vi "Help.About.vi"(11 "SW Version":T1={"AppName"="Automated Test Station", "Company"="Kwest Engineering", "Version"="v1.0.1", "Description"="1/25/2016"}) -> ()   [LabVIEW 2017]
uses:
  <vilib>/KATE/Module/Module.SW Version Info.ctl
  <vilib>/KATE/Module/Module Utils.lvlib
panel:
  in  "Close":bool
  out "About this Application:":string
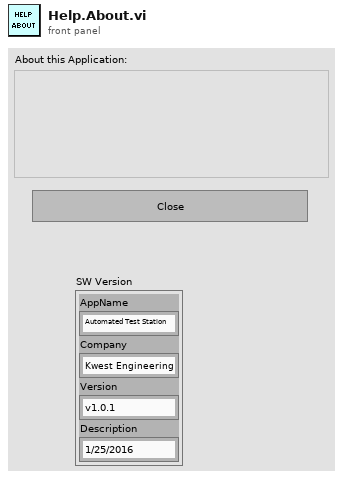
[diagram p1: front panel]
types:
  T1 = typedef "KATE_Lib.lvlib/Module Utils.lvlib/Module.SW Version Info.ctl" = cluster{"AppName":string, "Company":string, "Version":string, "Description":string}
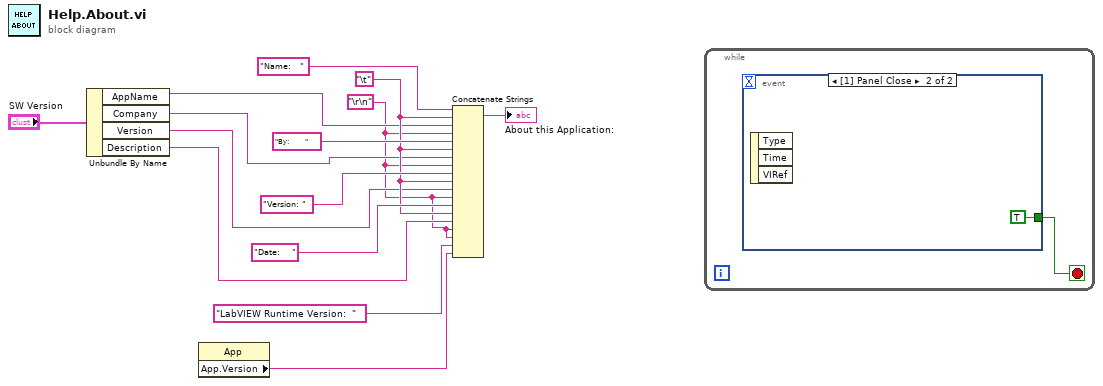
[diagram p0: block diagram]
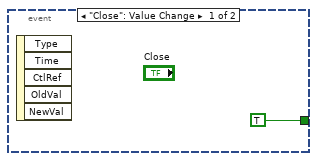
[diagram p2: hidden frame]
diagram:
  w3 = "\r\n"
  w9 = "\t"
  n1 = Unbundle By Name("SW Version") -> ("AppName"=w7:string, "Company"=w6:string, "Version"=w5:string, "Description"=w4:string)
  n2 = property class="App"() -> ("App.Version"=w1:string)  [unwired: 2 in, 2 out]
  n3 = Concatenate Strings("Name:   ", w9, w7, w3, "By:        ", w9, w6, w3, "Version: ", w9, w5, w3, "Date:    ", w9, w4, w3, w3, "LabVIEW Runtime Version:  ", w1) -> (→"About this Application:":string)
  n4 = while {
    stop <- w15 stop-if-true
    n5 = event shown="[1] Panel Close" {
      selector: _ -> [_ _]
      dyn-events: _ -> [_ _]
      timeout: _ -> [_ _]
      tunnel: [TRUE TRUE] -> w15
      event "Close": Value Change {
        n6 = event-data() -> ()  [unwired: 1 in, 5 out]
      }
      event Panel Close {
        n7 = event-data() -> ()  [unwired: 1 in, 3 out]
      }
    }
  }
